vi "Add Dither Noise.vi"(9 "amplitude (LSB)":dbl=1.0, 10 "bits":i32=24, 11 "Signal Properties":T1) -> (3 "Signal Properties":T1)   [LabVIEW 2021]
doc: "Adds dither noise of +/-1 LSB to the generated signal."
uses:
  <vilib>/PDM Acquisition Toolkit/host/Classes/Tasks/I2S Output/Control/SignalProperties.ctl
  <vilib>/PDM Acquisition Toolkit/host/Classes/Channels/I2S Ouput/Controls/GenerationChannelProperties.ctl
  <vilib>/PDM Acquisition Toolkit/host/Classes/Channels/I2S Ouput/I2S Output Channel.lvclass
  <vilib>/PDM Acquisition Toolkit/host/Classes/Tasks/I2S Output/I2S Output Task.lvclass
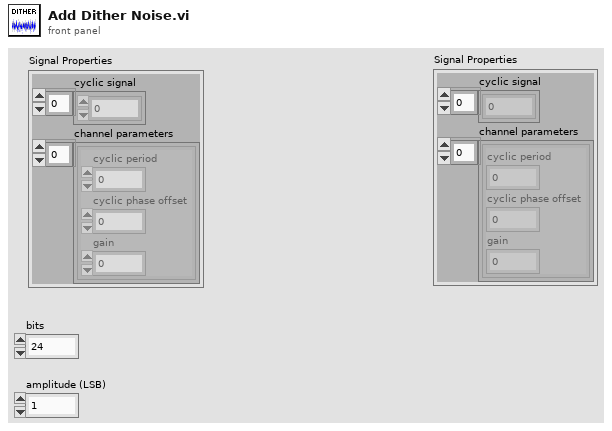
[diagram p1: front panel]
types:
  T1 = typedef "PDM Acquisition Class Library.lvlib/I2S Output Task.lvclass/SignalProperties.ctl" = cluster{"cyclic signal":dbl[], "channel parameters":T2[]}
  T2 = typedef "PDM Acquisition Class Library.lvlib/I2S Output Channel.lvclass/GenerationChannelProperties.ctl" = cluster{"cyclic period":dbl, "cyclic phase offset":dbl, "gain":dbl}
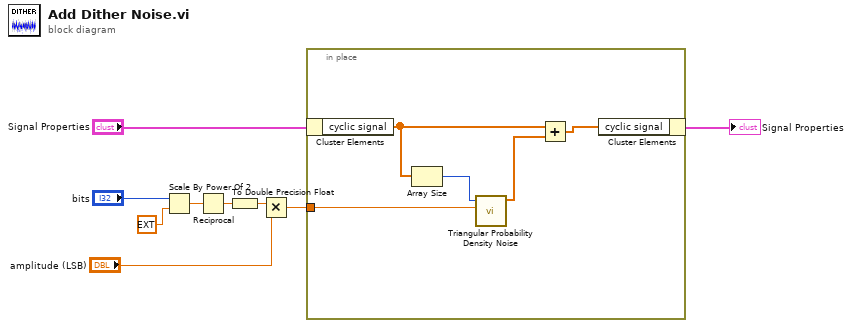
[diagram p0: block diagram]
diagram:
  n1 = Scale By Power Of 2(n="bits", x=ext 1.0) -> (x*2^n=w5:ext)
  n2 = Reciprocal(x=w5) -> (1/x=w2:ext)
  n3 = To Double Precision Float(number=w2) -> (double precision float=w1:dbl)
  n4 = Multiply(x=w1, y="amplitude (LSB)") -> (x*y=w4:dbl)
  n5 = in-place {
    in-place-border: w4 -> [w10]
    n6 = in-place-cluster #1("Signal Properties") -> ("cyclic signal"=w13:dbl[])
    n7 = Array Size(array=w13) -> (size(s)=w14:i32)
    n8 = call "Triangular Probability Density Noise.vi"("amplitude"=w10, "samples"=w14) -> ("TPDF noise"=w12:dbl[])  [unwired: 9 in]
    n9 = Add(x=w13, y=w12) -> (x+y=w11:dbl[])
    n10 = in-place-cluster #1("cyclic signal"=w11) -> (→"Signal Properties":T1)
  }
